vi "Flatten to CSV Record.vi"(7 "delimiter (,)":string=",", 10 "error in (no error)":errorcluster, 11 "row of strings":string[](array[string])) -> (2 "error out":errorcluster, 3 "CSV record":string, 5 "can be indented?":bool)   [LabVIEW 2013, in "infolib.lvlib"]
doc: "Convert 1D array of ANSI strings into a single CSV record (row).\n\nThe output CSV record string is formatted in accordance with RFC-4180 (see <b>http://tools.ietf.org/html/rfc4180<\\b>). \n\nAll cells containing double quotes (0x22), CR (0x0D) , LF (0x0A) or the delimiter character will be enclosed in double quotes. All double quote characters within a cell will be escaped using a second double quote character.\n\nRev. 0.0 2014-02-20 Ryan Porter\n- First Draft\n\nRev 0.1 2014-10-30 Ryan Porter\n- Convert all CRLF and CR within a cell to LF\n- Changed end of record to CRLF for compatibility with Excel CSV import/export\n\nRev 0.2 2017-01-03 modified for infolib"
uses:
  infolib.lvlib
panel:
  # "Flatten to CSV Record.vi\n\nConvert 1D array of ANSI strings into a single CSV record (row). The output CSV record string is formatted in accordance with RFC-4180 (see http://tools.ietf.org/html/rfc4180). \n\nAll cells containing double quotes (0x22), CR (0x0D) , LF (0x0A) or the delimiter character will be enclosed in double quotes. All double quote characters within a cell will be escaped using a second double quote character. A CRLF is appended to the end of the record."
  # "License: BSD (2-Clause) - http://opensource.org/licenses/BSD-2-Clause \n\nCopyright (c) 2014, Ryan Porter\nAll rights reserved."
  # "Robust CSV v1.1.0\n\nCopyright © 2014, Ryan Porter\nAll rights reserved.\n\nAuthor:\t Ryan Porter\nLAVA Name: Porter\nContact Info:\tContact via PM on lavag.org\n\nLabVIEW Versions:\nLV 2013 (Windows)\nLV 2012 (Windows)\nLV 8.6 (Windows)\n\nDependencies:\nLAVA Palette\n\nDescription:\nThis package contains VIs for reading and writing to CSV files that follow the CSV format outlined in RFC-4180 (see http://tools.ietf.org/html/rfc4180). Using this package, you can properly import CSV files that were exported from spreadsheet programs such as Microsoft Excel, Open Office or LibreOffice Calc as well as export CSV files that will be compatible with any program capable of interpreting CSV files.\n \nThis implementation of the CSV format is capable of handling escaped fields such as those containing commas (or other field delimiters), multiple lines, and double quotes.\n\nInstallation and instructions:\nInstall VIP package using JKI VI Package Manager.\n\nExamples:\n\"<LabVIEW>\\examples\\LAVA\\Robust CSV\\Robust CSV Example Usage.vi\"\tDemonstrates usage of the Read CSV and Write CSV file.\n\nKnown Issues:\nnone\n\nAcknowledgements:\nPhillip Brooks: \"Parse CSV String.vi\" is a modified version of his \"CSV Data File Parser.vi\". His method of parsing the CSV string was much more efficient than my original implementation.\n\nVersion History:\nv1.0.0: Initial release of the code.\nv1.0.1: Modified \"Flatten to CSV Record.vi\" to play nice with Excel CSV import when multi-line cells are present.\nv1.1.0: Moved to LAVA palette & built to VI package file.\n\nLicense:\nDistributed under the BSD 2-Clause (http://opensource.org/licenses/BSD-2-Clause)\nSee link for a full description of the license.\n\nSupport:\nIf you have any problems with this code or want to suggest features go to lavag.org and Navigate to LAVA > Resources > Code Repository (Certified) and\nsearch for the \"Robust CSV\" support page. Or try this link: http://lavag.org/files/file/239-robust-csv/\n\nDistribution:\nThis code was downloaded from the LAVA Code Repository found at lavag.org"
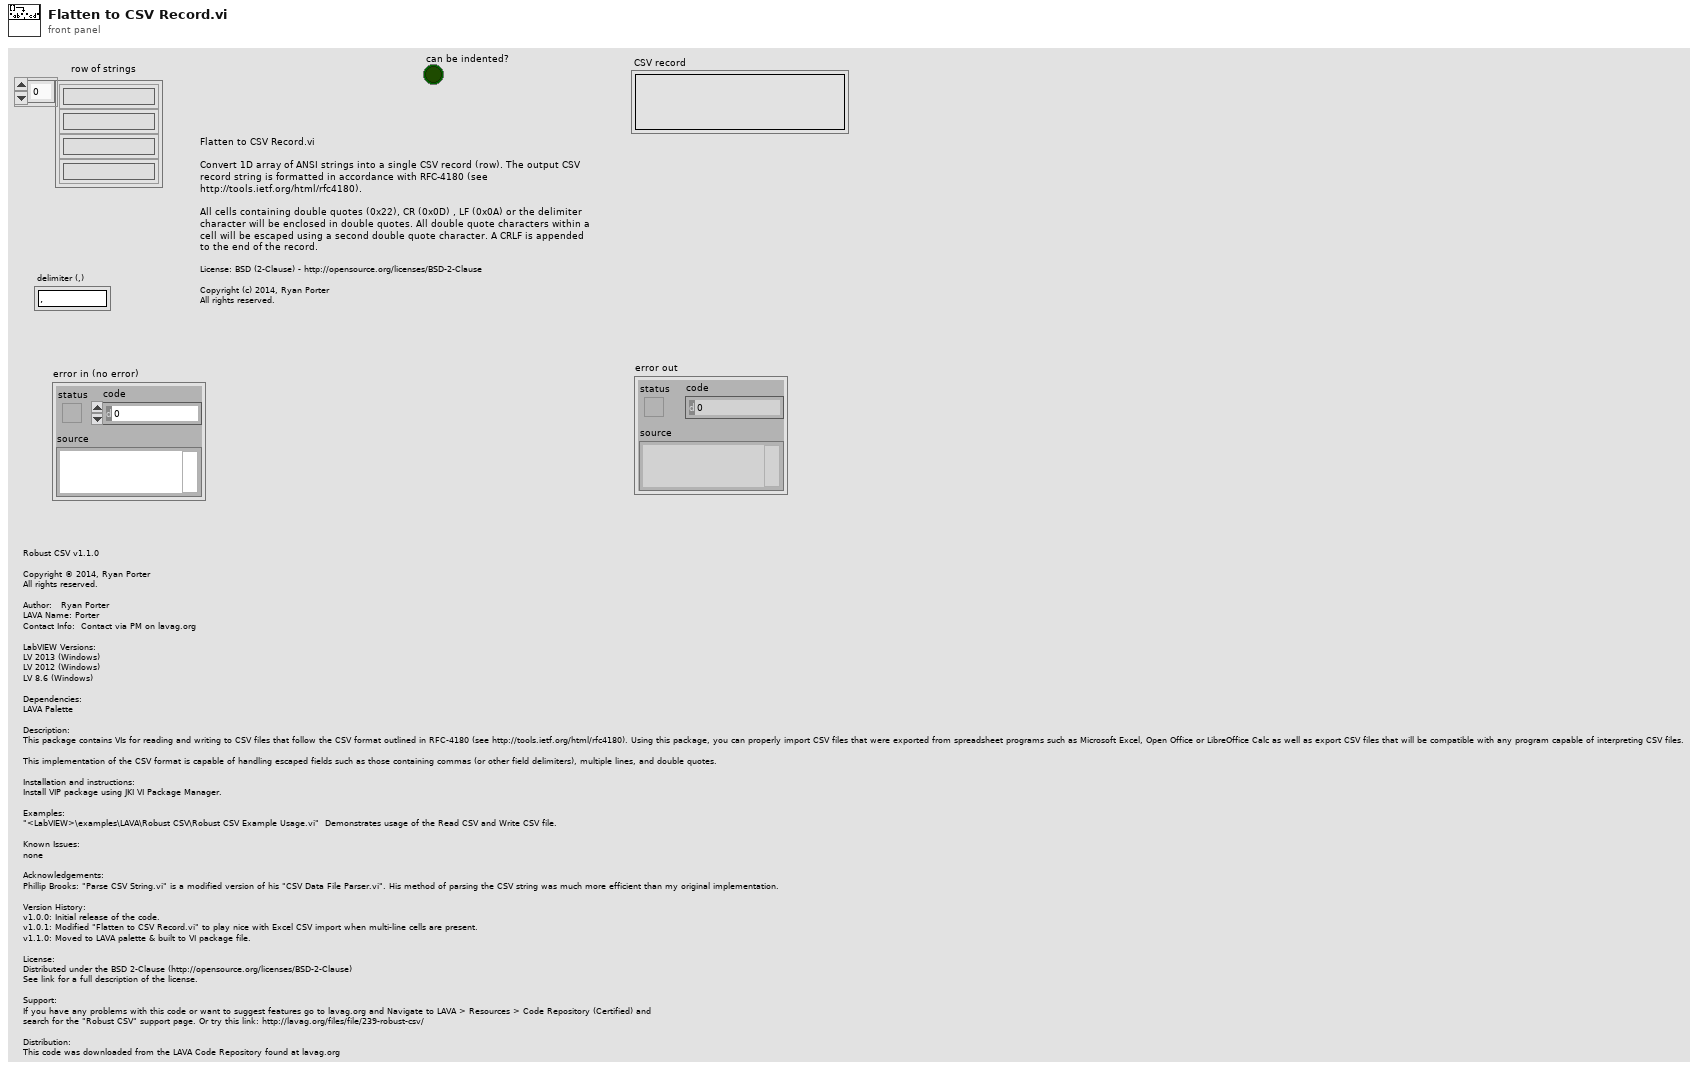
[diagram p1: front panel]
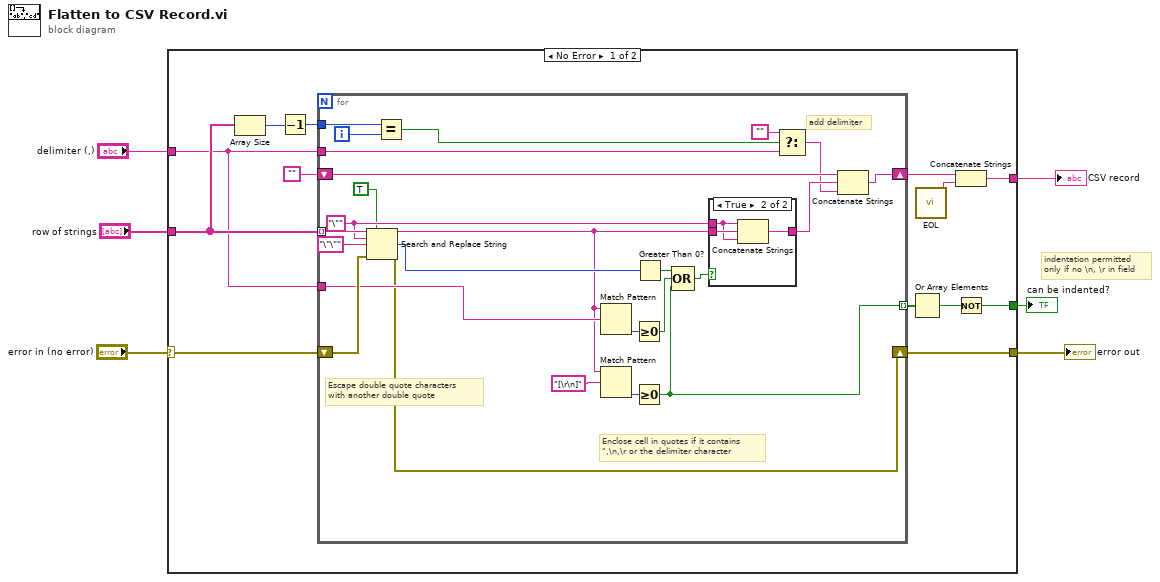
[diagram p0: block diagram]
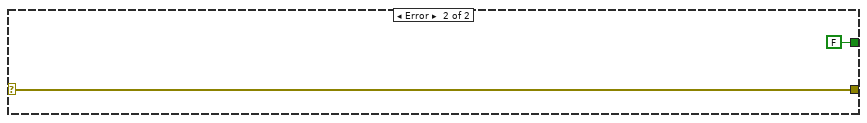
[diagram p3: hidden frame]
diagram:
  # "indentation permitted\nonly if no \\n, \\r in field"
  n1 = case shown="No Error" "error in (no error)" {
    selector: "error in (no error)" -> [w13 w50]
    tunnel: "row of strings" -> [w17 _]
    tunnel: "delimiter (,)" -> [w10 _]
    tunnel: [w14 _] -> w4
    tunnel: [w12 w50] -> w2
    tunnel: [w7 FALSE] -> w1
    frame No Error {
      n2 = Array Size(array=w17) -> (size(s)=w16:i32)
      n3 = Decrement(x=w16) -> (x-1=w18:i32)
      n4 = for {
        tunnel: w17 -> [w44] mode=indexing
        shift-right: [w41] -> w15
        shift-left: "" -> [w40]
        tunnel: w10 -> [w35]
        tunnel: w18 -> [w32]
        shift-right: [w23] -> w12
        shift-left: w13 -> [w29]
        tunnel: [w20] -> w11 mode=indexing
        tunnel: w10 -> [w24]
        i -> [w37]
        w42 = "\"" ("search string")
        # "Escape double quote characters\nwith another double quote"
        # "Enclose cell in quotes if it contains\n\",\\n,\\r or the delimiter character"
        # "add delimiter"
        n5 = Search and Replace String(replace all?=TRUE ("replace all? (F)"), input string=w44, search string=w42, replace string="\"\"" ("replace string (\"\")"), error in=w29) -> (result string=w22:string, number of replacements=w31:i32, error out=w23:errorcluster)  [unwired: 4 out]
        n6 = Equal?(x=w32, y=w37) -> (x = y?=w36:bool)
        n7 = Match Pattern(string=w22, regular expression=w24) -> (offset past match=w38:i32)  [unwired: 4 out]
        n8 = Match Pattern(string=w22, regular expression="[\r\n]") -> (offset past match=w26:i32)  [unwired: 4 out]
        n9 = Greater Or Equal To 0?(x=w38) -> (x >= 0?=w21:bool)
        n10 = Greater Or Equal To 0?(x=w26) -> (x >= 0?=w20:bool)
        n11 = Greater Than 0?(x=w31) -> (x > 0?=w27:bool)
        n12 = Compound Arithmetic op=OR(w27, w21, w20) -> (w30:bool)
        n13 = case shown="True" w30 {
          tunnel: w22 -> [w45 w48]
          tunnel: w42 -> [_ w47]
          tunnel: [w45 w46] -> w39
          frame False {
          }
          frame True {
            n14 = Concatenate Strings(w47, w48, w47) -> (w46:string)
          }
        }
        n15 = Select(t="", s=w36, f=w35) -> (s? t:f=w33:string)
        n16 = Concatenate Strings(w40, w39, w33) -> (w41:string)
      }
      n17 = Or Array Elements(Boolean array=w11) -> (logical OR=w8:bool)
      n18 = call "EOL.vi"() -> ("eol"=w9:string)  [unwired: 11 in]
      n19 = Concatenate Strings(w15, w9) -> (w14:string)
      n20 = Not(x=w8) -> (.not. x?=w7:bool)
    }
    frame Error {
    }
  }
  "CSV record" <- w4
  "error out" <- w2
  "can be indented?" <- w1
